vi "OpenBase.vi"(5 "LogEnabled":bool, 7 "LogPath":path, 8 "error in (no error)":errorcluster, 9 "Instance":string, 10 "BaudRate":u32=125000, 11 "Konvolucio MCAN120803 Adapter Class in":refnum<class "Konvolucio MCAN120803 Adapter Class.lvclass">) -> (0 "error out":errorcluster, 3 "Konvolucio MCAN120803 Adapter Class out":refnum<class "Konvolucio MCAN120803 Adapter Class.lvclass">)   [LabVIEW 2011, in "Konvolucio MCAN120803 Adapter Class.lvclass"]
uses:
  Konvolucio MCAN120803 Adapter Class.lvclass
  Konvolucio MCAN120803 Adapter Class.lvclass/Konvolucio MCAN120803 Adapter Class.ctl
  <instrlib>/Konvolucio MCAN120803/Konvolucio MCAN120803.lvlib
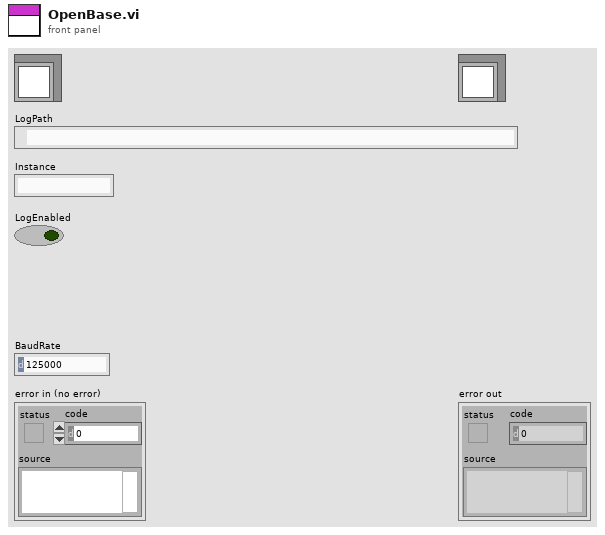
[diagram p1: front panel]
types:
  T1 = typedef "Konvolucio MCAN120803.lvlib/CanHandleType.ctl" = cluster{"AdapterDevice":refnum<k24>}
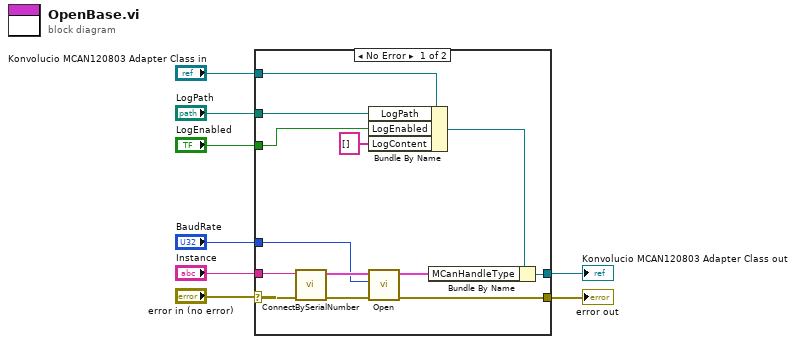
[diagram p0: block diagram]
diagram:
  n1 = case shown="No Error" "error in (no error)" {
    selector: "error in (no error)" -> [w16 w23]
    tunnel: [w18 w23] -> w7
    tunnel: "Konvolucio MCAN120803 Adapter Class in" -> [w21 w22]
    tunnel: "LogPath" -> [w20 _]
    tunnel: "LogEnabled" -> [w19 _]
    tunnel: "BaudRate" -> [w13 _]
    tunnel: [w10 w22] -> w2
    tunnel: "Instance" -> [w15 _]
    frame No Error {
      n2 = call <instrlib>:"ConnectBySerialNumber.vi"("error in"=w16, "AdapterSerialNumber"=w15) -> ("error out"=w17:errorcluster, "CanHandleOut"=w14:T1)  [unwired: 8 in]
      n3 = Bundle By Name(cluster=w21, "LogPath"=w20, "LogEnabled"=w19, "LogContent"=string[] []) -> (w12:refnum<class "Konvolucio MCAN120803 Adapter Class.lvclass">)
      n4 = call <instrlib>:"Open.vi"("error in"=w17, "Baudrate"=w13, "CanHandleIn"=w14) -> ("error out"=w18:errorcluster, "CanHandleOut"=w11:T1)  [unwired: 7 in]
      n5 = Bundle By Name(cluster=w12, "MCanHandleType"=w11) -> (w10:refnum<class "Konvolucio MCAN120803 Adapter Class.lvclass">)
    }
    frame Error {
    }
  }
  "error out" <- w7
  "Konvolucio MCAN120803 Adapter Class out" <- w2
